vi "Fetch Measurement (Harmonic).vi"(0 "VISA resource name":refnum<visa-resource-name>, 5 "Timeout (10000 ms)":i32=10000 format="%.0g", 7 "Fetch Option (1)":i32=1, 9 "Data Type (0:Total Harmonic Distortion)":i32(ring) items=["Total Harmonic Distortion", "Frequency", "Specified Harmonic Amplitude"], 11 "error in (no error)":errorcluster) -> (4 "VISA resource name out":refnum<visa-resource-name>, 6 "Measurement Data":dbl[](array[numeric]), 15 "error out":errorcluster)   [LabVIEW 2018, in "Agilent MXA Series.lvlib"]
doc: "Returns the results of last harmonic measurement and does not initiate data acquisition.\n\n<B>Note:</B>\n\nUse this VI only with other low-level VIs. The high-level VIs automatically incorporate this functionality. This VI does not check the instrument status."
uses:
  Agilent MXA Series.lvlib
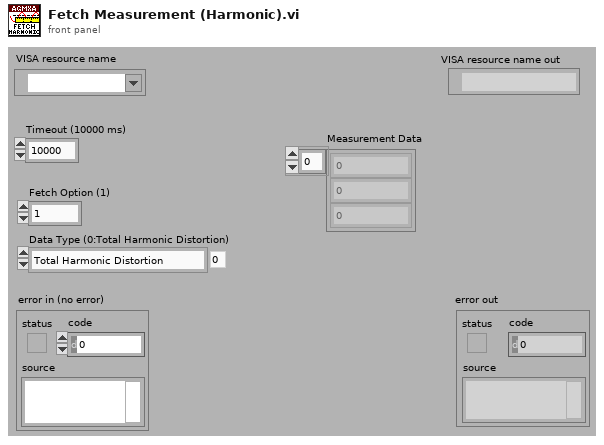
[diagram p1: front panel]
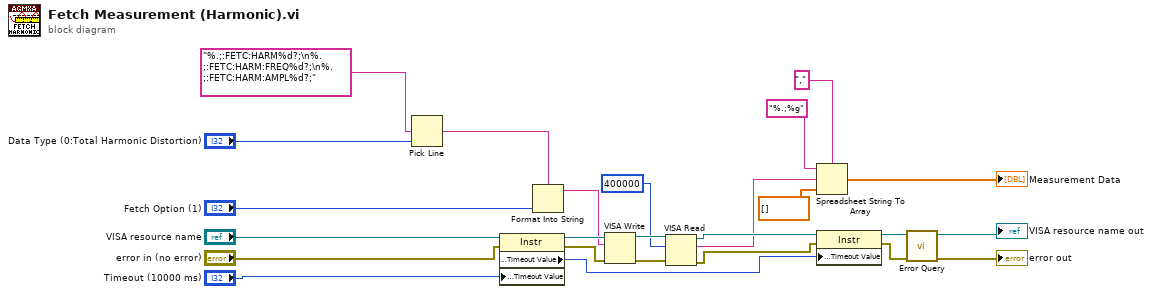
[diagram p0: block diagram]
diagram:
  n1 = Pick Line(multi-line string="%.;:FETC:HARM%d?;\n%.;:FETC:HARM:FREQ%d?;\n%.;:FETC:HARM:AMPL%d?;", line index="Data Type (0:Total Harmonic Distortion)") -> (output string=w1:string)  [unwired: 1 in]
  n2 = property on="Property Node" class="Instr"(reference="VISA resource name", error in="error in (no error)", "General Settings:Timeout Value"="Timeout (10000 ms)") -> (reference out=w23:refnum<visa-resource-name>, error out=w24:errorcluster, "General Settings:Timeout Value"=w18:u32)
  n3 = Format Into String(format string=w1, "Fetch Option (1)") -> (resulting string=w6:string)  [unwired: 2 in, 1 out]
  n4 = VISA Write(VISA resource name=w23, write buffer=w6, error in (no error)=w24) -> (VISA resource name out=w21:refnum<visa-resource-name>, error out=w22:errorcluster)  [unwired: 1 out]
  n5 = VISA Read(VISA resource name=w21, byte count=400000, error in (no error)=w22) -> (VISA resource name out=w20:refnum<visa-resource-name>, read buffer=w14:string, error out=w19:errorcluster)  [unwired: 1 out]
  n6 = Spreadsheet String To Array(delimiter (Tab)=",", format string="%.;%g", spreadsheet string=w14, array type (2D Dbl)=dbl[] [] ("Measurement Data 2")) -> (array=→"Measurement Data":dbl[])
  n7 = property on="Property Node" class="Instr"(reference=w20, error in=w19, "General Settings:Timeout Value"=w18) -> (reference out=w9:refnum<visa-resource-name>, error out=w10:errorcluster)
  n8 = call "Error Query.vi"("error in (no error)"=w10, "VISA resource name"=w9) -> ("error out"=→"error out":errorcluster, "VISA resource name out"=→"VISA resource name out":refnum<visa-resource-name>)  [unwired: 6 in, 2 out]
